vi "ConvertByteArrayToGDSII8ByteReal.vi"(11 "Data":u8[](array[numeric])=[62, 65, 137, 55, 75, 198, 167, 244, 57, 68, 184, 47, 160, 155, 90, 88]) -> (3 "Array of Values":dbl[](array[numeric]))   [LabVIEW 2019]
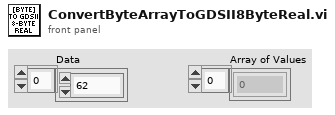
[diagram p1: front panel]
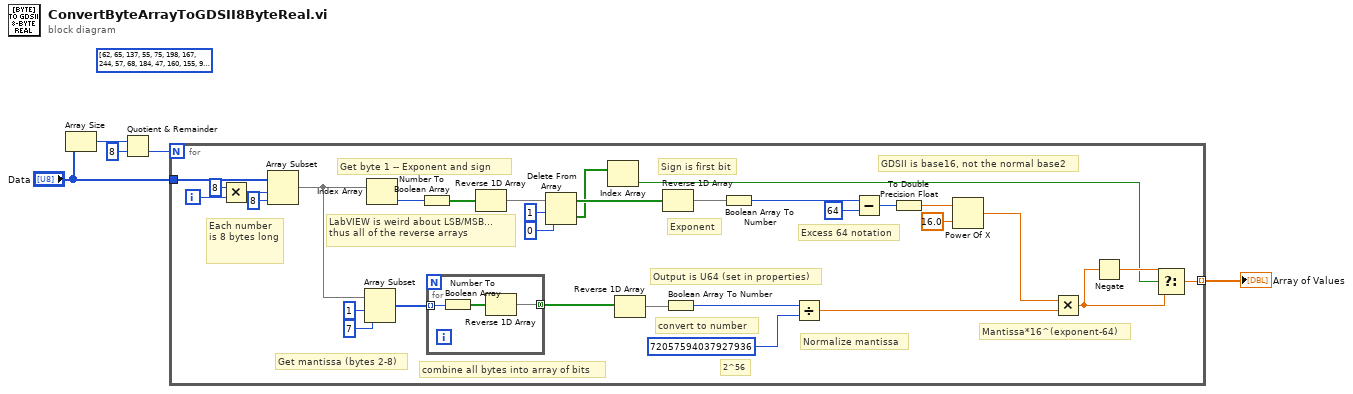
[diagram p0: block diagram]
diagram:
  (unwired) u8[] [62, 65, 137, 55, 75, 198, 167, 244, 57, 68, 184, 47, 160, 155, 90, 88] ("Data")
  n1 = Array Size(array="Data") -> (size(s)=w1:i32)
  n2 = Quotient & Remainder(x=w1, y=8) -> (floor(x/y)=w3:i32)  [unwired: 1 out]
  n3 = for {
    N: w3 -> [_]
    tunnel: [w12] -> w2 mode=indexing
    tunnel: "Data" -> [w10]
    i -> [w7]
    # "combine all bytes into array of bits"
    # "LabVIEW is weird about LSB/MSB... thus all of the reverse arrays"
    # "Get mantissa (bytes 2-8)"
    # "Mantissa*16^(exponent-64)"
    # "GDSII is base16, not the normal base2"
    # "Excess 64 notation"
    # "convert to number"
    # "Normalize mantissa"
    # "Exponent"
    # "Sign is first bit"
    # "Get byte 1 -- Exponent and sign"
    # "Each number is 8 bytes long"
    # "2^56"
    # "Output is U64 (set in properties)"
    n4 = Multiply(x=8, y=w7) -> (x*y=w9:i32)
    n5 = Array Subset(array=w10, index=w9, length=8) -> (w11:u8[])
    n6 = Array Subset(array=w11, index=1, length=7) -> (w29:u8[])
    n7 = Index Array(array=w11) -> (element=w37:u8)  [unwired: 1 in]
    n8 = Number To Boolean Array(number=w37) -> (Boolean array=w36:bool[])
    n9 = for {
      tunnel: w29 -> [w40] mode=indexing
      tunnel: [w38] -> w28 mode=concatenating
      n10 = Number To Boolean Array(number=w40) -> (Boolean array=w39:bool[])
      n11 = Reverse 1D Array(array=w39) -> (reversed array=w38:bool[])
    }
    n12 = Reverse 1D Array(array=w36) -> (reversed array=w32:bool[])
    n13 = Delete From Array(array=w32, length=1, index=0) -> (deleted portion=w17:bool[], array with subset deleted=w33:bool[])
    n14 = Index Array(array=w17) -> (element=w15:bool)  [unwired: 1 in]
    n15 = Reverse 1D Array(array=w28) -> (reversed array=w27:bool[])
    n16 = Reverse 1D Array(array=w33) -> (reversed array=w13:bool[])
    n17 = Boolean Array To Number(Boolean array=w27) -> (number=w26:u64)
    n18 = Boolean Array To Number(Boolean array=w13) -> (number=w25:i32)
    n19 = Divide(x=w26, y=u64 72057594037927936) -> (x/y=w22:dbl)
    n20 = Subtract(x=w25, y=64) -> (x-y=w19:i32)
    n21 = To Double Precision Float(number=w19) -> (double precision float=w18:dbl)
    n22 = Power Of X(1:16.0 ("x"), 2:w18) -> (0:w21:dbl)
    n23 = Multiply(x=w21, y=w22) -> (x*y=w14:dbl)
    n24 = Negate(x=w14) -> (-x=w16:dbl)
    n25 = Select(t=w16, s=w15, f=w14) -> (s? t:f=w12:dbl)
  }
  "Array of Values" <- w2
